vi "切割.vi"() -> ()   [LabVIEW 2010]
uses:
  <vilib>/Instr/_visa.llb/VISA Configure Serial Port (Instr).vi
panel:
  in  "切割程序":enum32{"参数设定", "速度设定", "程序设定"}(tab)
  in  "VISA resource name":refnum<visa-resource-name>="COM1"
  in  "X轴速度mm/s":dbl(knob) scale=0.0..100.0
  in  "Y轴速度mm/s":dbl(knob) scale=0.0..100.0
  in  "布尔":bool
  in  "确认":bool
  in  "X边长（mm）":dbl
  in  "Y边长（mm）":dbl
  in  "圈数":i32
  out "进度条":dbl(slide) scale=0.0..100.0
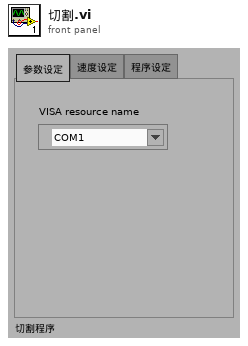
[diagram p1: front panel]
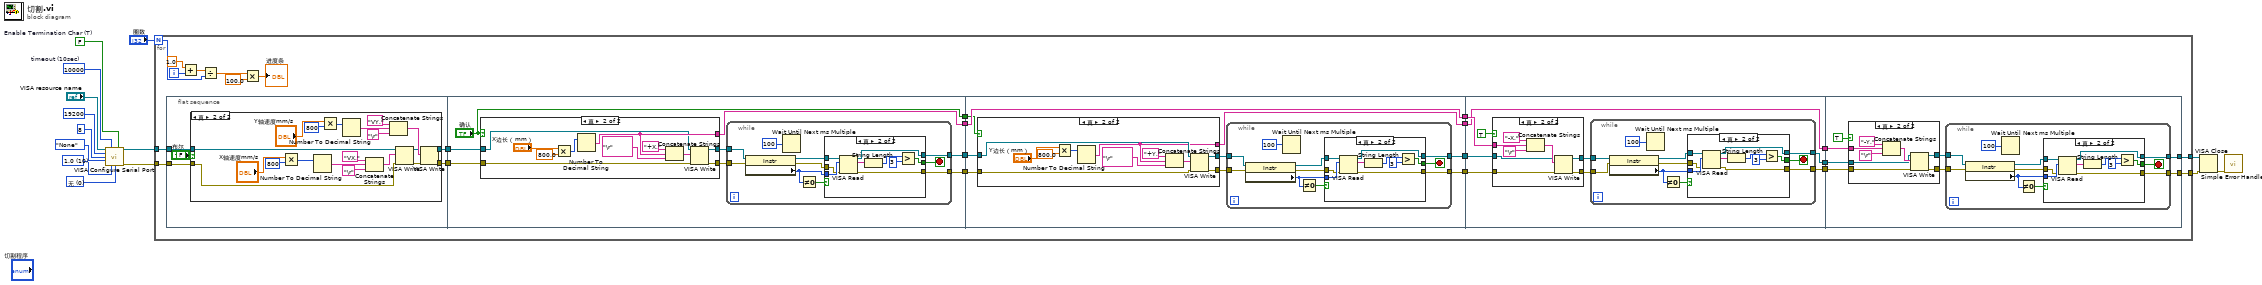
[diagram p0: block diagram]
diagram:
  w1 = u16 0 items=["无", "XON/XOFF", "RTS/CTS", "XON/XOFF & RTS/CTS", "DTR/DSR", "XON/XOFF & DTR/DSR"] ("flow control (0:none)")
  w2 = u16 10 items=["1.0"=10, "1.5"=15, "2.0"=20] ("stop bits (10: 1 bit)")
  w12 = FALSE  # Enable Termination Char (T)
  w13 = u32 10000  # timeout (10sec)
  n1 = call-poly "VISA Configure Serial Port"("VISA resource name"="VISA resource name", "timeout (10sec)"=w13, "Enable Termination\nChar (T)"=w12, "baud rate (9600)"=u32 19200, "data bits (8)"=u16 8, "parity (0:none)"=enum16{"None", "Odd", "Even", "Mark", "Space"}."None", "stop bits (10: 1 bit)"=w2, "flow control (0:none)"=w1) -> ("VISA resource name out"=w11:refnum<visa-resource-name>, "error out"=w10:errorcluster)  [unwired: 1 in, 5 out]
  n2 = for {
    N: "圈数" -> [w23]
    tunnel: w11 -> [w38]
    tunnel: w10 -> [w35]
    tunnel: [w25] -> w8
    tunnel: [w24] -> w7
    i -> [w18]
    n3 = flat-sequence {
      tunnel: w35 -> [w42]
      tunnel: w38 -> [w43]
      tunnel: [w41] -> w16
      tunnel: [w40] -> w15
      tunnel: [w71] -> w37
      tunnel: [w70] -> w36
      tunnel: [w69] -> w31
      tunnel: ["确认"] -> w26
      tunnel: w16 -> [w67]
      tunnel: w15 -> [w66]
      tunnel: w37 -> [w110]
      tunnel: w36 -> [w109]
      tunnel: [w108] -> w34
      tunnel: [w107] -> w33
      tunnel: [w106] -> w32
      tunnel: w31 -> [w106]
      tunnel: [w105] -> w27
      tunnel: w26 -> [w104]
      tunnel: w34 -> [w149]
      tunnel: w33 -> [w148]
      tunnel: w32 -> [w147]
      tunnel: [w146] -> w30
      tunnel: [w145] -> w29
      tunnel: [w144] -> w28
      tunnel: w27 -> [w144]
      tunnel: w30 -> [w184]
      tunnel: w29 -> [w183]
      tunnel: w28 -> [w182]
      tunnel: [w180] -> w25
      tunnel: [w179] -> w24
      frame #0 {
        n4 = case shown="真" FALSE {
          tunnel: w43 -> [w45 w59]
          tunnel: w42 -> [w44 w49]
          tunnel: [w45 w47] -> w41
          tunnel: [w44 w46] -> w40
          frame False {
          }
          frame True {
            n5 = Multiply ("乘")(x="X轴速度mm/s", y=u16 800) -> (x*y=w63:u16)
            n6 = Number To Decimal String(number=w63) -> (decimal integer string=w62:string)  [unwired: 1 out]
            n7 = Multiply ("乘")(x="Y轴速度mm/s", y=u16 800) -> (x*y=w55:u16)
            n8 = Number To Decimal String(number=w55) -> (decimal integer string=w54:string)  [unwired: 1 out]
            n9 = Concatenate Strings("VX," ("字符串"), w62, "\r" ("字符串")) -> (w58:string)
            n10 = Concatenate Strings("VY," ("字符串"), w54, "\r" ("字符串")) -> (w51:string)
            n11 = VISA Write(VISA resource name=w59, write buffer=w58, error in (no error)=w49) -> (VISA resource name out=w50:refnum<visa-resource-name>, error out=w48:errorcluster)  [unwired: 1 out]
            n12 = VISA Write(VISA resource name=w50, write buffer=w51, error in (no error)=w48) -> (VISA resource name out=w47:refnum<visa-resource-name>, error out=w46:errorcluster)  [unwired: 1 out]
          }
        }
      }
      frame #1 {
        n13 = case shown="真" "确认" {
          tunnel: [_ w103] -> w72
          tunnel: [_ w102] -> w73
          tunnel: [_ w96] -> w69
          tunnel: w67 -> [_ w94]
          tunnel: w66 -> [_ w93]
          frame False {
          }
          frame True {
            n14 = Multiply ("乘")(x="X边长（mm）", y=800.0) -> (x*y=w99:u16)
            n15 = Number To Decimal String(number=w99) -> (decimal integer string=w96:string)  [unwired: 1 out]
            n16 = Concatenate Strings("+X," ("字符串"), w96, "\r" ("字符串")) -> (w97:string)
            n17 = VISA Write(VISA resource name=w94, write buffer=w97, error in (no error)=w93) -> (VISA resource name out=w102:refnum<visa-resource-name>, error out=w103:errorcluster)  [unwired: 1 out]
          }
        }
        n18 = while {
          tunnel: w73 -> [w82]
          tunnel: w72 -> [w81]
          tunnel: [w76] -> w71
          tunnel: [w75] -> w70
          stop <- w74 stop-if-true
          n19 = property class="Instr"(reference=w82, error in=w81) -> (reference out=w83:refnum<visa-resource-name>, error out=w80:errorcluster, "Serial Settings:Number of Bytes at Serial Port"=w78:u32)
          n20 = Wait Until Next ms Multiple(millisecond multiple=u32 100 ("毫秒倍数")) -> ()  [unwired: 1 out]
          n21 = Not Equal To 0?(x=w78) -> (x != 0?=w77:bool)
          n22 = case shown="真" w77 {
            tunnel: w83 -> [_ w92]
            tunnel: w78 -> [_ w91]
            tunnel: w80 -> [_ w90]
            tunnel: [_ w89] -> w76
            tunnel: [_ w88] -> w75
            tunnel: [_ w84] -> w74
            frame False {
            }
            frame True {
              n23 = VISA Read(VISA resource name=w92, byte count=w91, error in (no error)=w90) -> (VISA resource name out=w89:refnum<visa-resource-name>, read buffer=w87:string, error out=w88:errorcluster)  [unwired: 1 out]
              n24 = String Length(string=w87) -> (length=w86:i32)
              n25 = Greater?(x=w86, y=3) -> (0:w84:bool)
            }
          }
        }
      }
      frame #2 {
        n26 = case shown="真" w104 {
          tunnel: [_ w123] -> w111
          tunnel: [_ w122] -> w112
          tunnel: w110 -> [_ w116]
          tunnel: w109 -> [_ w115]
          tunnel: [_ w114] -> w105
          frame False {
          }
          frame True {
            n27 = Multiply ("乘")(x="Y边长（mm）", y=800.0) -> (x*y=w119:u16)
            n28 = Number To Decimal String(number=w119) -> (decimal integer string=w114:string)  [unwired: 1 out]
            n29 = Concatenate Strings("+Y," ("字符串"), w114, "\r" ("字符串")) -> (w117:string)
            n30 = VISA Write(VISA resource name=w116, write buffer=w117, error in (no error)=w115) -> (VISA resource name out=w122:refnum<visa-resource-name>, error out=w123:errorcluster)  [unwired: 1 out]
          }
        }
        n31 = while {
          tunnel: [w128] -> w108
          tunnel: [w127] -> w107
          tunnel: w112 -> [w126]
          tunnel: w111 -> [w125]
          stop <- w124 stop-if-true
          n32 = property class="Instr"(reference=w126, error in=w125) -> (reference out=w133:refnum<visa-resource-name>, error out=w132:errorcluster, "Serial Settings:Number of Bytes at Serial Port"=w130:u32)
          n33 = Wait Until Next ms Multiple(millisecond multiple=u32 100 ("毫秒倍数")) -> ()  [unwired: 1 out]
          n34 = Not Equal To 0?(x=w130) -> (x != 0?=w129:bool)
          n35 = case shown="真" w129 {
            tunnel: w133 -> [_ w142]
            tunnel: w130 -> [_ w141]
            tunnel: w132 -> [_ w140]
            tunnel: [_ w139] -> w128
            tunnel: [_ w138] -> w127
            tunnel: [_ w134] -> w124
            frame False {
            }
            frame True {
              n36 = VISA Read(VISA resource name=w142, byte count=w141, error in (no error)=w140) -> (VISA resource name out=w139:refnum<visa-resource-name>, read buffer=w137:string, error out=w138:errorcluster)  [unwired: 1 out]
              n37 = String Length(string=w137) -> (length=w135:i32)
              n38 = Greater?(x=w135, y=3) -> (0:w134:bool)
            }
          }
        }
      }
      frame #3 {
        n39 = case shown="真" TRUE {
          tunnel: [_ w159] -> w150
          tunnel: [_ w158] -> w151
          tunnel: w149 -> [_ w154]
          tunnel: w148 -> [_ w153]
          tunnel: w147 -> [_ w152]
          frame False {
          }
          frame True {
            n40 = Concatenate Strings("-X," ("字符串"), w152, "\r" ("字符串")) -> (w155:string)
            n41 = VISA Write(VISA resource name=w154, write buffer=w155, error in (no error)=w153) -> (VISA resource name out=w158:refnum<visa-resource-name>, error out=w159:errorcluster)  [unwired: 1 out]
          }
        }
        n42 = while {
          tunnel: [w164] -> w146
          tunnel: [w163] -> w145
          tunnel: w151 -> [w162]
          tunnel: w150 -> [w161]
          stop <- w160 stop-if-true
          n43 = property class="Instr"(reference=w162, error in=w161) -> (reference out=w169:refnum<visa-resource-name>, error out=w168:errorcluster, "Serial Settings:Number of Bytes at Serial Port"=w166:u32)
          n44 = Wait Until Next ms Multiple(millisecond multiple=u32 100 ("毫秒倍数")) -> ()  [unwired: 1 out]
          n45 = Not Equal To 0?(x=w166) -> (x != 0?=w165:bool)
          n46 = case shown="真" w165 {
            tunnel: w169 -> [_ w178]
            tunnel: w166 -> [_ w177]
            tunnel: w168 -> [_ w176]
            tunnel: [_ w175] -> w164
            tunnel: [_ w174] -> w163
            tunnel: [_ w170] -> w160
            frame False {
            }
            frame True {
              n47 = VISA Read(VISA resource name=w178, byte count=w177, error in (no error)=w176) -> (VISA resource name out=w175:refnum<visa-resource-name>, read buffer=w173:string, error out=w174:errorcluster)  [unwired: 1 out]
              n48 = String Length(string=w173) -> (length=w171:i32)
              n49 = Greater?(x=w171, y=3) -> (0:w170:bool)
            }
          }
        }
      }
      frame #4 {
        n50 = case shown="真" TRUE {
          tunnel: [_ w194] -> w185
          tunnel: [_ w193] -> w186
          tunnel: w184 -> [_ w189]
          tunnel: w183 -> [_ w188]
          tunnel: w182 -> [_ w187]
          frame False {
          }
          frame True {
            n51 = Concatenate Strings("-Y," ("字符串"), w187, "\r" ("字符串")) -> (w190:string)
            n52 = VISA Write(VISA resource name=w189, write buffer=w190, error in (no error)=w188) -> (VISA resource name out=w193:refnum<visa-resource-name>, error out=w194:errorcluster)  [unwired: 1 out]
          }
        }
        n53 = while {
          tunnel: [w199] -> w180
          tunnel: [w198] -> w179
          tunnel: w186 -> [w197]
          tunnel: w185 -> [w196]
          stop <- w195 stop-if-true
          n54 = property class="Instr"(reference=w197, error in=w196) -> (reference out=w204:refnum<visa-resource-name>, error out=w203:errorcluster, "Serial Settings:Number of Bytes at Serial Port"=w201:u32)
          n55 = Wait Until Next ms Multiple(millisecond multiple=u32 100 ("毫秒倍数")) -> ()  [unwired: 1 out]
          n56 = Not Equal To 0?(x=w201) -> (x != 0?=w200:bool)
          n57 = case shown="真" w200 {
            tunnel: w204 -> [_ w213]
            tunnel: w201 -> [_ w212]
            tunnel: w203 -> [_ w211]
            tunnel: [_ w210] -> w199
            tunnel: [_ w209] -> w198
            tunnel: [_ w205] -> w195
            frame False {
            }
            frame True {
              n58 = VISA Read(VISA resource name=w213, byte count=w212, error in (no error)=w211) -> (VISA resource name out=w210:refnum<visa-resource-name>, read buffer=w208:string, error out=w209:errorcluster)  [unwired: 1 out]
              n59 = String Length(string=w208) -> (length=w206:i32)
              n60 = Greater?(x=w206, y=3) -> (0:w205:bool)
            }
          }
        }
      }
    }
    n61 = Add(x=1.0, y=w18) -> (x+y=w17:dbl)
    n62 = Divide(x=w17, y=w23) -> (x/y=w22:dbl)
    n63 = Multiply(x=w22, y=100.0) -> (x*y=→"进度条":dbl)
  }
  n64 = VISA Close(VISA resource name=w8, error in (no error)=w7) -> (error out=w9:errorcluster)
  n65 = call <vilib>:"Simple Error Handler.vi"("error in (no error)"=w9) -> ()  [unwired: 1 in, 8 out]
